vi "HEWH Get FHD.vi"(7 "Water Heater Type":T1, 8 "error in (no error)":errorcluster, 10 "FHD During 1 Hour Input":T2 {"Data Indexes"."15 sec after Draw Index" format="%#.2f"; "Data Indexes"."15 sec after Draw Timestamp" format="%#.2f"; "Data Indexes"."Test Start Timestamp" format="%.2f"; "Data Indexes"."Test End Timestamp" format="%.2f"; "Data Indexes"."T0 Timestamp" format="%.2f"; "Data Indexes"."Tsf Timestamp" format="%.2f"; "Data Indexes"."Tsu0 Timestamp" format="%.2f"; "Data Indexes"."Tmax1 Timestamp" format="%.2f"; "Data Indexes"."Draw Index Timestamp" format="%#.2f"; "Data Indexes"."Non-Draw Timestamp" format="%#.2f"; "Data Indexes"."Heating Timestamp" format="%#.2f"; "Data Indexes"."Start Energy (BTU-Gas)" format="%.6f"; "Data Indexes"."Start Watt Hours" format="%.6f"; "Static Data"."V - Volume of Wh (True)" format="%.5f"; "Static Data"."T-Ambinet Nominal (°F)" format="%.5f"; "Static Data"."T-Inlet Setpoint (°F)" format="%.5f"; "Static Data"."T-Wh Setpoint (°F)" format="%.5f"; "Sampled Data"."Qe (Wh)" format="%.5f"; "Sampled Data"."Tau stby2 (hr)" format="%.5f"; "Sampled Data"."Tastby2 (°F)" format="%.5f"; "Sampled Data"."Qf (BTU)" format="%.5f"; "Sampled Data"."Qe (BTU)" format="%.5f"; "Sampled Data"."Tmax1 (°F)" format="%.5f"; "Sampled Data"."T0 (°F)" format="%.5f"; "Sampled Data"."Qr (BTU)" format="%.5f"; "Sampled Data"."T 24(°F)" format="%.5f"; "Sampled Data"."T astby(°F)" format="%.5f"; "Sampled Data"."T tstby(°F)" format="%.5f"; "Sampled Data"."T su0(°F)" format="%.5f"; "Sampled Data"."T suf(°F)" format="%.5f"; "Sampled Data"."Tau stby_1 (hr)" format="%.5f"; "Sampled Data"."Qsuf (BTU)" format="%.5f"; "Sampled Data"."Qsu0 (BTU)" format="%.5f"; "Calculated Values"."Draw Bonus Volume (gal)" format="%.6f"; "Calculated Values"."Adjustment Factor" format="%.6f"; "Calculated Values"."T*avg_del(n-1)" format="%.6f"; "Calculated Values"."T*min(n-1)" format="%.6f"; "Calculated Values"."T*avg_del(n)" format="%.6f"; "Calculated Values"."Vn" format="%.6f"; "Calculated Values"."Qdm (BTU)" format="%.6f"; "Calculated Values"."QHWD (BTU)" format="%.6f"; "Calculated Values"."QHW (BTU)" format="%.6f"; "Calculated Values"."UEF" format="%.6f"; "Calculated Values"."QHW67 (BTU)" format="%.6f"; "Calculated Values"."Qda (BTU)" format="%.6f"; "Calculated Values"."Qd (BTU)" format="%.6f"; "Calculated Values"."Q (BTU)" format="%.6f"; "Calculated Values"."UA (BTU/(hr*F))" format="%.6f"; "Calculated Values"."Qhr (BTU/hr)" format="%.6f"; "Calculated Values"."Qstby (BTU)" format="%.6f"; "Calculated Values"."nu_r" format="%.6f"; "Calculated Values"."CpUEF (BTU/(lb*F))" format="%.6f"; "Calculated Values"."rho_nu (lb/gal)" format="%.6f"; "Calculated Values"."V1- Vol (Gal)" format="%.6f"; "Calculated Values"."M cluster mass removed (lb)" format="%.6f"; "Calculated Values"."Cp theoretical (BTU/(lbm °F))" format="%.6f"; "Calculated Values"."Tin1 - Mean Inlet 1st Cluster (°F)" format="%.6f"; "Calculated Values"."Tdel1-Mean Outlet 1st Cluster(°F)" format="%.6f"; "Calculated Values"."Cp 24 (BTU/(lb*F))" format="%.6f"; "Calculated Values"."Cp standby (BTU/(lb*F))" format="%.6f"; "Calculated Values"."Cp2 (BTU/(lb*F))" format="%.6f"; "Calculated Values"."Cp1 (BTU/(lb*F))" format="%.6f"; "Calculated Values"."rho 24 (lb/gal)" format="%.6f"; "Calculated Values"."rho standby (lb/gal)" format="%.6f"; "Calculated Values"."rho 2 (lb/gal)" format="%.6f"; "Calculated Values"."Density of cold water All (lbm/gal)" format="%#.3g"; "Calculated Values"."CpHW (BTU/(lbm °F))" format="%#.3g"; "Calculated Values"."Density of hot water All (lbm/gal)" format="%#.3g"; "Calculated Values"."Mass of water All (lbm)" format="%#.3f"}, 11 "1st Hour Location":path) -> (0 "error out":errorcluster, 1 "First Hour Rating (Gallons)":dbl, 2 "FHD During 1 Hour Output":T2={"Calculated Values"={"Draw Cluster - Actual (Gal)"=[], "Mass of water All (lbm)"=[], "Density of hot water All (lbm/gal)"=[], "CpHW (BTU/(lbm °F))"=[], "rho 2 (lb/gal)"=0.0, "rho standby (lb/gal)"=0.0, "rho 24 (lb/gal)"=0.0, "Cp1 (BTU/(lb*F))"=0.0, "Cp2 (BTU/(lb*F))"=0.0, "Cp standby (BTU/(lb*F))"=0.0, "Cp 24 (BTU/(lb*F))"=0.0, "nu_r"=0.0, "Qstby (BTU)"=0.0, "Qhr (BTU/hr)"=0.0, "UA (BTU/(hr*F))"=0.0, "Q (BTU)"=0.0, "Qd (BTU)"=0.0, "Qda (BTU)"=0.0, "QHW67 (BTU)"=0.0, "UEF"=0.0, "Tdel1-Mean Outlet 1st Cluster(°F)"=0.0, "Tin1 - Mean Inlet 1st Cluster (°F)"=0.0, "Cp theoretical (BTU/(lbm °F))"=0.0, "M cluster mass removed (lb)"=0.0, "V1- Vol (Gal)"=0.0, "Test Data -Start to End (Full Index)"=[], "rho_nu (lb/gal)"=0.0, "Density of cold water All (lbm/gal)"=[], "CpUEF (BTU/(lb*F))"=0.0, "QHW (BTU)"=0.0, "QHWD (BTU)"=0.0, "Qdm (BTU)"=0.0, "FHD-After 1 Hour (String)"=[], "Vn"=0.0, "T*avg_del(n)"=0.0, "Max Location"=0, "T*min(n-1)"=0.0, "T*avg_del(n-1)"=0.0, "Temp Greater than T*min(n-1)"=FALSE, "Adjustment Factor"=0.0, "Draw Bonus Volume (gal)"=0.0, "Flow Type - End Condition"=enum."ForcedDrawAfterHour"}, "Sampled Data"={"Cold Water Draw Amounts-(Gal)"=[14.98, 1.97, 9.0, 8.97, 4.98, 0.98, 0.96, 0.96, 0.96, 1.96, 1.99, 6.98], "T del_all - Outlet Temps (°F)"=[121.5, 121.3, 124.5, 120.0, 121.2, 120.1, 119.0, 120.3, 116.6, 118.8, 118.3, 118.3], "T in_all - Inlet Temps (°F)"=[58.5, 58.2, 58.4, 58.6, 58.6, 58.1, 58.1, 58.3, 56.3, 58.5, 58.5, 58.5], "Qsu0 (BTU)"=9772.3, "Qsuf (BTU)"=9773.0, "Tau stby_1 (hr)"=6.7, "T suf(°F)"=107.7, "T su0(°F)"=109.3, "T tstby(°F)"=108.5, "T astby(°F)"=68.2, "T 24(°F)"=117.9, "Qr (BTU)"=7628.5, "T0 (°F)"=121.1, "Tmax1 (°F)"=122.4, "Qe (BTU)"=29606.3, "Qf (BTU)"=0.0, "Tastby2 (°F)"=68.3, "RTD Out Full Data\nSet (Each Draw)"=[], "RTD IN Full Data\nSet (Each Draw)"=[], "Tau stby2 (hr)"=23.406, "Hot Water Draw Amounts-(Gal)"=[], "Cold Flow Rate (GPM)"=[], "Hot Flow Rate (GPM)"=[], "Softw Elapsed Time\n Full Data Set (Each Draw)"=[], "Cold Gal Total Full\nData Set (Each Draw)"=[], "Total Hot Draw Amount (Gal) "=0.0, "Total Cold Draw Amount (Gal)"=0.0, "Qe (Wh)"=0.0, "Hot Gal Total Full\nData Set (Each Draw)"=[]}, "Static Data"={"T-Wh Setpoint (°F)"=125.0, "T-Inlet Setpoint (°F)"=58.0, "T-Ambinet Nominal (°F)"=67.5, "V - Volume of Wh (True)"=46.0}, "Data Indexes"={"Test Start-Full Index (Found)"=0, "Header Length"=0, "Draw Index (Found)"=[], "Nr"=0, "Start Watt Hours"=0.0, "Tsu0 Index (Found)"=0, "Tsf Index (Found)"=0, "Start Energy (BTU-Gas)"=0.0, "Draws in Cluster"=0, "T0 Index-Full Index (Found)"=0, "Non-Draw Index (Found)"=[], "Tmax1 Index (Found)"=0, "Test End-Full Index (Found)"=0, "Heating Index (Found)"=[], "Heating Timestamp"=[], "Non-Draw Timestamp"=[], "Draw Index Timestamp"=[], "Tmax1 Timestamp"=0.0, "Tsu0 Timestamp"=0.0, "Tsf Timestamp"=0.0, "T0 Timestamp"=0.0, "Test End Timestamp"=0.0, "Test Start Timestamp"=0.0, "15 sec after Draw Timestamp"=[], "15 sec after Draw Index"=[], "Tmax1 Occurred During a Draw"=FALSE, "FHD Total Time (Sec)"=0.0, "Draw Pattern"=enum."Very Small Usage", "Standby Valid"=FALSE}, "Raw Data"={"Elapsed Time Index (DBL)"=0, "Software Elapsed Time Index (DBL)"=0, "TC Tree Avg Index (DBL)"=0, "Watt Hours -Wh Index (DBL)"=0, "Energy BTU Index (DBL)"=0, "Totalized Flow Index (DBL)"=0, "Flow Rate Index (DBL)"=0, "Program Status Index (Str)"=0, "RTDin Index (DBL)"=0, "RTDout Index (DBL)"=0, "RTDamb Index (DBL)"=0, "Test Data-Start to End DBL"=[], "Data Type"=enum."GEA Inlet Side Meter", "Heat Source Index (DBL)"=0, "Hot Water Rate GPM (DBL)"=0, "Hot Water Total - GAL (DBL)"=0, "FHD-After 1 hour"=[], "Humidity -% RH (DBL)"=0, "Voltage - V (DBL)"=0, "Draw Count (DBL)"=0, "Elapsed Time Index (Str)"=0, "Software Elapsed Time Index (Str)"=0, "Frequency-Hz (Str)"=0, "RTDin Index (Str)"=0, "RTDout Index (Str)"=0, "RTDamb Index (Str)"=0, "UE (Str)"=0, "LE (Str)"=0, "Compressor (Str)"=0, "Flow Rate Index (Str)"=0, "Hot Water Total - GAL (Str)"=0}, "Tolerance Check (T)=Pass"={"Flow Rate"=FALSE, "Totalized Flow"=FALSE, "Ambient Temp (Full Range)"=FALSE, "Ambient Humidity (Full Range)"=FALSE, "Inlet Temp"=FALSE, "Outlet Temp"=FALSE, "Valid Test"=FALSE, "Individual Totalized Flow"=FALSE, "Data Sheet Check"="", "Inlet Temperature"=[], "Tinlet Max"=[], "Tinlet Min"=[], "Flow Rate Max (Tol)"=[], "Flow Rate Min (Tol)"=[], "Amb Temp Max"=0.0, "Amb Temp Min"=0.0, "Toutlet Max - Draw 1"=0.0, "Humidity Upper Tolerance (%)"=0.0, "Total Volume Tolerance (Gal)"=0.0, "Humidity Lower Tolerance (%)"=0.0, "Flow Rate Max\nPer Draw"=[], "Flow Rate Min\nPer Draw"=[], "Ambient Humidity (Runtime)"=FALSE, "Humidity Avg (Runtime)"=0.0, "Ambient Temp (On-Time AVG)"=FALSE, "Ambient Temp (Off-Time AVG)"=FALSE, "Amb Temp OFF Avg"=0.0, "Amb Temp ON Avg"=0.0, "Voltage (Heating)"=FALSE, "Voltage (Min)"=0.0, "Voltage (Max)"=0.0, "Toutlet Max"=[], "Toutlet Min"=[], "Test_Avg_Outlet_Temp"=0.0}, "Test Information"={"TR Number"="", "Lab ID"="", "Notes/Config"="", "Model Number"="", "Serial Number"="", "Lab Technician"="", "Engineer"="", "Type of Fuel"="", "Samp Received Date"="", "Samp Test Date"="", "Report Date"="", "Rate Input (kW or BTU/hr)"="", "Measured Input (kW or BTU/hr)"="", "Filename"="", "Calibration Information"=[], "Calculator Version"="", "Minimum UEF Per CFR"=0.0, "UEF Report Information"=[], "FHR Report Information"=[], "FHR Front Panel Display"=[], "UEF Front Panel Display"=[], "Draw Outlet Temp Viewer"=[]}} {"Data Indexes"."15 sec after Draw Index" format="%#.2f"; "Data Indexes"."15 sec after Draw Timestamp" format="%#.2f"; "Data Indexes"."Test Start Timestamp" format="%.2f"; "Data Indexes"."Test End Timestamp" format="%.2f"; "Data Indexes"."T0 Timestamp" format="%.2f"; "Data Indexes"."Tsf Timestamp" format="%.2f"; "Data Indexes"."Tsu0 Timestamp" format="%.2f"; "Data Indexes"."Tmax1 Timestamp" format="%.2f"; "Data Indexes"."Draw Index Timestamp" format="%#.2f"; "Data Indexes"."Non-Draw Timestamp" format="%#.2f"; "Data Indexes"."Heating Timestamp" format="%#.2f"; "Data Indexes"."Start Energy (BTU-Gas)" format="%.6f"; "Data Indexes"."Start Watt Hours" format="%.6f"; "Static Data"."V - Volume of Wh (True)" format="%.5f"; "Static Data"."T-Ambinet Nominal (°F)" format="%.5f"; "Static Data"."T-Inlet Setpoint (°F)" format="%.5f"; "Static Data"."T-Wh Setpoint (°F)" format="%.5f"; "Sampled Data"."Qe (Wh)" format="%.5f"; "Sampled Data"."Tau stby2 (hr)" format="%.5f"; "Sampled Data"."Tastby2 (°F)" format="%.5f"; "Sampled Data"."Qf (BTU)" format="%.5f"; "Sampled Data"."Qe (BTU)" format="%.5f"; "Sampled Data"."Tmax1 (°F)" format="%.5f"; "Sampled Data"."T0 (°F)" format="%.5f"; "Sampled Data"."Qr (BTU)" format="%.5f"; "Sampled Data"."T 24(°F)" format="%.5f"; "Sampled Data"."T astby(°F)" format="%.5f"; "Sampled Data"."T tstby(°F)" format="%.5f"; "Sampled Data"."T su0(°F)" format="%.5f"; "Sampled Data"."T suf(°F)" format="%.5f"; "Sampled Data"."Tau stby_1 (hr)" format="%.5f"; "Sampled Data"."Qsuf (BTU)" format="%.5f"; "Sampled Data"."Qsu0 (BTU)" format="%.5f"; "Calculated Values"."Draw Bonus Volume (gal)" format="%.6f"; "Calculated Values"."Adjustment Factor" format="%.6f"; "Calculated Values"."T*avg_del(n-1)" format="%.6f"; "Calculated Values"."T*min(n-1)" format="%.6f"; "Calculated Values"."T*avg_del(n)" format="%.6f"; "Calculated Values"."Vn" format="%.6f"; "Calculated Values"."Qdm (BTU)" format="%.6f"; "Calculated Values"."QHWD (BTU)" format="%.6f"; "Calculated Values"."QHW (BTU)" format="%.6f"; "Calculated Values"."UEF" format="%.6f"; "Calculated Values"."QHW67 (BTU)" format="%.6f"; "Calculated Values"."Qda (BTU)" format="%.6f"; "Calculated Values"."Qd (BTU)" format="%.6f"; "Calculated Values"."Q (BTU)" format="%.6f"; "Calculated Values"."UA (BTU/(hr*F))" format="%.6f"; "Calculated Values"."Qhr (BTU/hr)" format="%.6f"; "Calculated Values"."Qstby (BTU)" format="%.6f"; "Calculated Values"."nu_r" format="%.6f"; "Calculated Values"."CpUEF (BTU/(lb*F))" format="%.6f"; "Calculated Values"."rho_nu (lb/gal)" format="%.6f"; "Calculated Values"."V1- Vol (Gal)" format="%.6f"; "Calculated Values"."M cluster mass removed (lb)" format="%.6f"; "Calculated Values"."Cp theoretical (BTU/(lbm °F))" format="%.6f"; "Calculated Values"."Tin1 - Mean Inlet 1st Cluster (°F)" format="%.6f"; "Calculated Values"."Tdel1-Mean Outlet 1st Cluster(°F)" format="%.6f"; "Calculated Values"."Cp 24 (BTU/(lb*F))" format="%.6f"; "Calculated Values"."Cp standby (BTU/(lb*F))" format="%.6f"; "Calculated Values"."Cp2 (BTU/(lb*F))" format="%.6f"; "Calculated Values"."Cp1 (BTU/(lb*F))" format="%.6f"; "Calculated Values"."rho 24 (lb/gal)" format="%.6f"; "Calculated Values"."rho standby (lb/gal)" format="%.6f"; "Calculated Values"."rho 2 (lb/gal)" format="%.6f"; "Calculated Values"."Density of cold water All (lbm/gal)" format="%#.3g"; "Calculated Values"."CpHW (BTU/(lbm °F))" format="%#.3g"; "Calculated Values"."Density of hot water All (lbm/gal)" format="%#.3g"; "Calculated Values"."Mass of water All (lbm)" format="%#.3f"}, 4 "FHD Full Data":string[][](array[string]), 6 "PercentInRange":dbl)   [LabVIEW 2023]
uses:
  Type Definitions/UEF Constants.ctl
  Type Definitions/HEWH Draw Stats.ctl
  Type Definitions/HEWH FHR Draw Type.ctl
  Type Definitions/FHR Bins.ctl
  Type Definitions/HEWH Meter Type.ctl
  Type Definitions/HEWH Water Heater Type.ctl
  Type Definitions/HEWH Test Type.ctl
  Type Definitions/HEWH Index Type.ctl
  <vilib>/Utility/file.llb/Read Delimited Spreadsheet (string).vi
  <vilib>/Utility/file.llb/Read Delimited Spreadsheet (DBL).vi
panel:
  # "FHR"
  # "FHR"
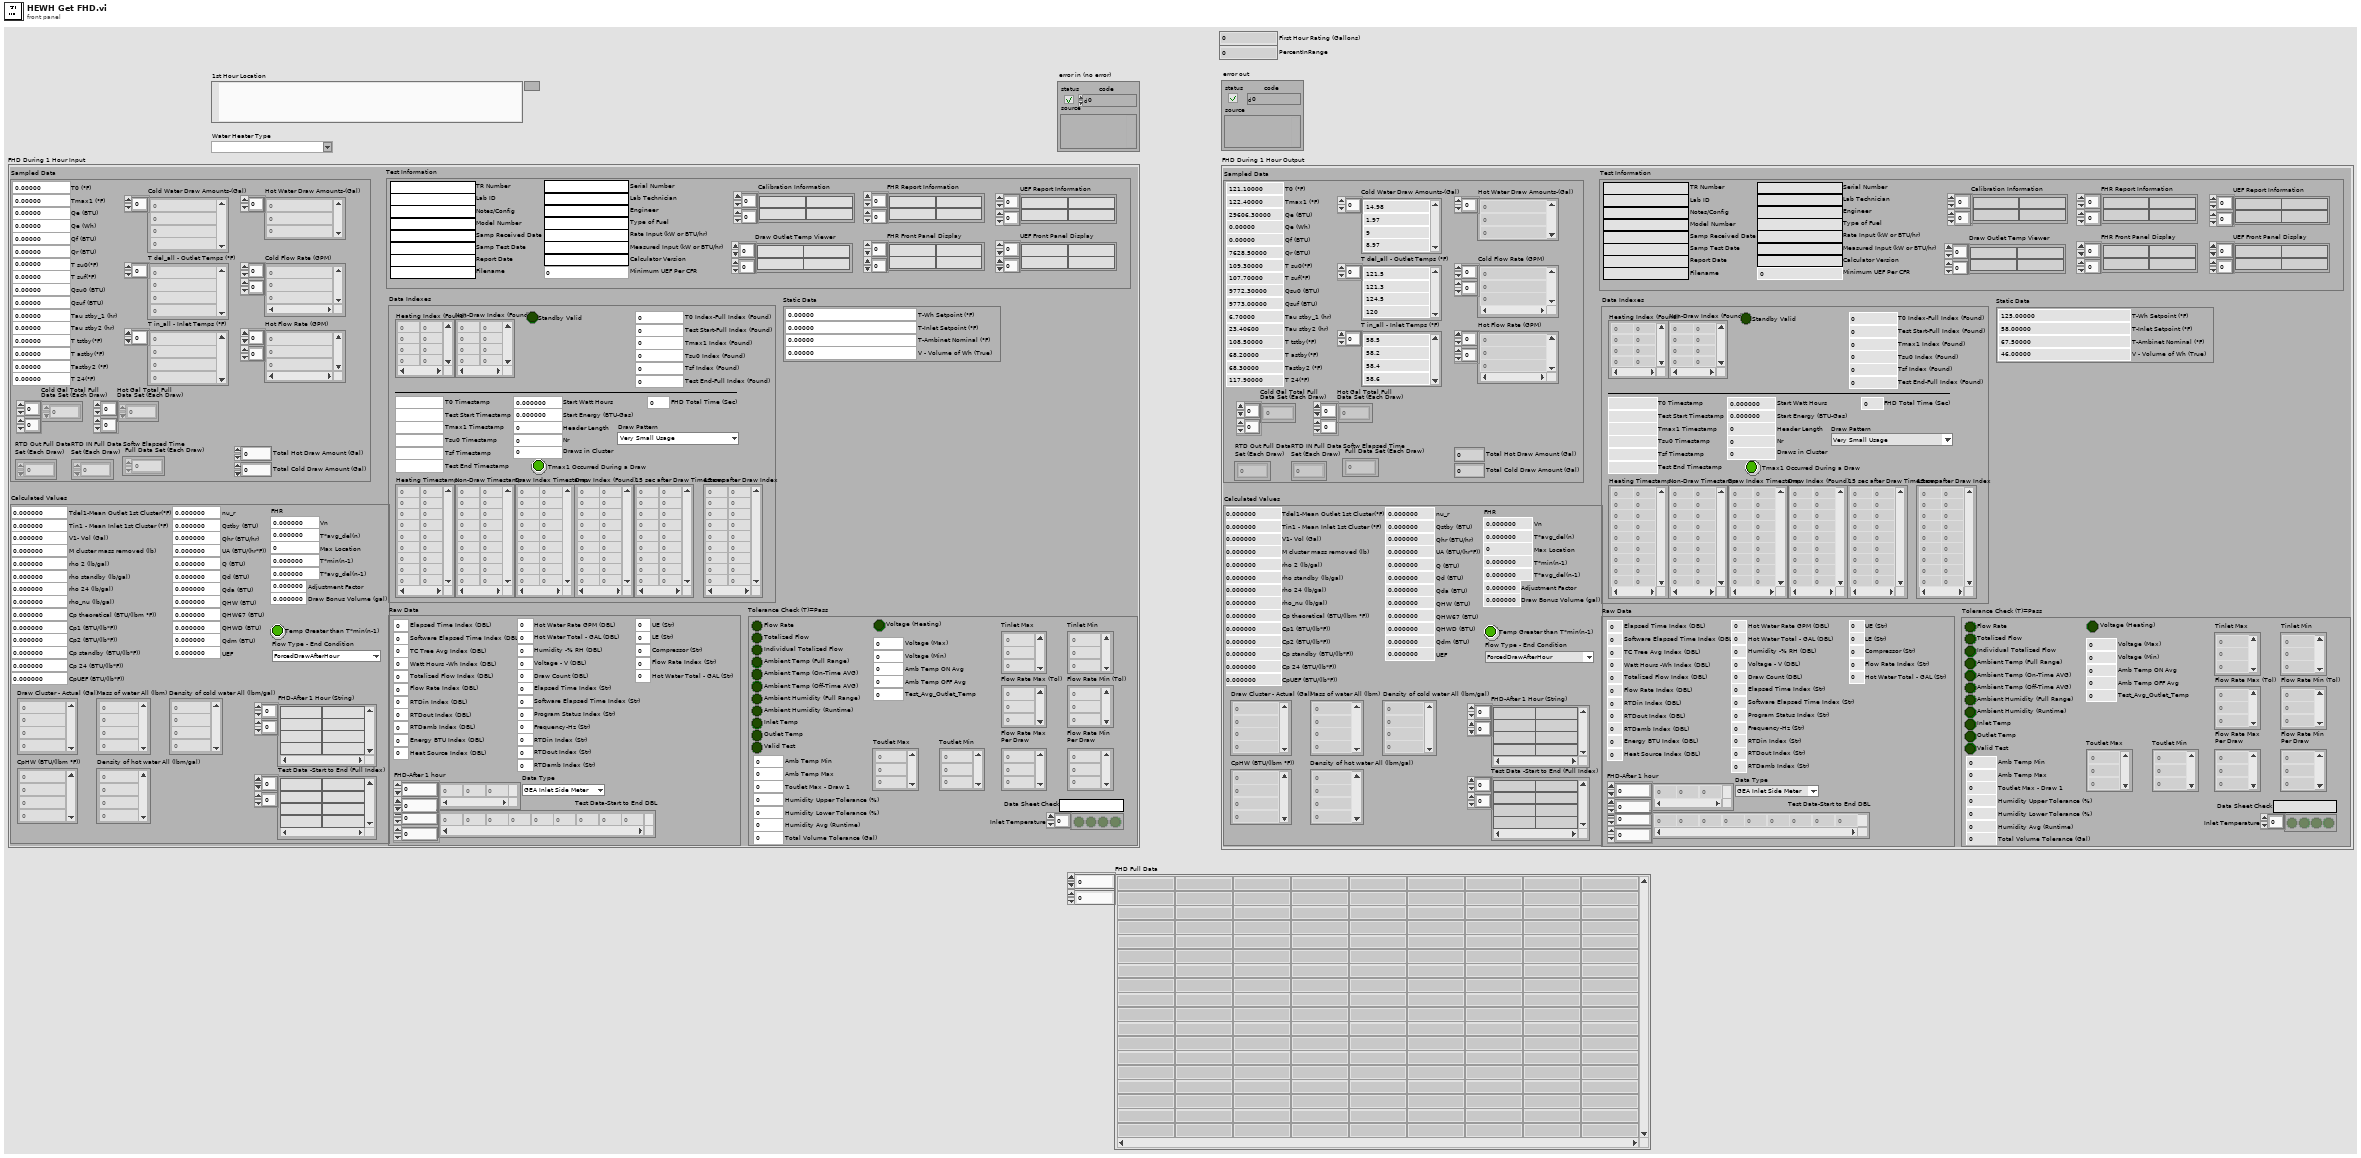
[diagram p1: front panel]
types:
  T1 = typedef "HEWH Water Heater Type.ctl" = string
  T2 = typedef "UEF Constants.ctl" = cluster{"Calculated Values":T3, "Sampled Data":cluster{"Cold Water Draw Amounts-(Gal)":dbl[], "T del_all - Outlet Temps (°F)":dbl[], "T in_all - Inlet Temps (°F)":dbl[], "Qsu0 (BTU)":dbl, "Qsuf (BTU)":dbl, "Tau stby_1 (hr)":dbl, "T suf(°F)":dbl, "T su0(°F)":dbl, "T tstby(°F)":dbl, "T astby(°F)":dbl, "T 24(°F)":dbl, "Qr (BTU)":dbl, "T0 (°F)":dbl, "Tmax1 (°F)":dbl, "Qe (BTU)":dbl, "Qf (BTU)":dbl, "Tastby2 (°F)":dbl, "RTD Out Full Data\nSet (Each Draw)":dbl[][], "RTD IN Full Data\nSet (Each Draw)":dbl[][], "Tau stby2 (hr)":dbl, "Hot Water Draw Amounts-(Gal)":dbl[], "Cold Flow Rate (GPM)":dbl[][], "Hot Flow Rate (GPM)":dbl[][], "Softw Elapsed Time\n Full Data Set (Each Draw)":dbl[][], "Cold Gal Total Full\nData Set (Each Draw)":dbl[][], "Total Hot Draw Amount (Gal) ":dbl, "Total Cold Draw Amount (Gal)":dbl, "Qe (Wh)":dbl, "Hot Gal Total Full\nData Set (Each Draw)":dbl[][]}, "Static Data":cluster{"T-Wh Setpoint (°F)":dbl, "T-Inlet Setpoint (°F)":dbl, "T-Ambinet Nominal (°F)":dbl, "V - Volume of Wh (True)":dbl}, "Data Indexes":cluster{"Test Start-Full Index (Found)":i32, "Header Length":i32, "Draw Index (Found)":i32[][], "Nr":i32, "Start Watt Hours":dbl, "Tsu0 Index (Found)":i32, "Tsf Index (Found)":i32, "Start Energy (BTU-Gas)":dbl, "Draws in Cluster":i32, "T0 Index-Full Index (Found)":i32, "Non-Draw Index (Found)":i32[][], "Tmax1 Index (Found)":i32, "Test End-Full Index (Found)":i32, "Heating Index (Found)":i32[][], "Heating Timestamp":dbl[][], "Non-Draw Timestamp":dbl[][], "Draw Index Timestamp":dbl[][], "Tmax1 Timestamp":dbl, "Tsu0 Timestamp":dbl, "Tsf Timestamp":dbl, "T0 Timestamp":dbl, "Test End Timestamp":dbl, "Test Start Timestamp":dbl, "15 sec after Draw Timestamp":dbl[][], "15 sec after Draw Index":dbl[][], "Tmax1 Occurred During a Draw":bool, "FHD Total Time (Sec)":dbl, "Draw Pattern":T5, "Standby Valid":bool}, "Raw Data":cluster{"Elapsed Time Index (DBL)":i32, "Software Elapsed Time Index (DBL)":i32, "TC Tree Avg Index (DBL)":i32, "Watt Hours -Wh Index (DBL)":i32, "Energy BTU Index (DBL)":i32, "Totalized Flow Index (DBL)":i32, "Flow Rate Index (DBL)":i32, "Program Status Index (Str)":i32, "RTDin Index (DBL)":i32, "RTDout Index (DBL)":i32, "RTDamb Index (DBL)":i32, "Test Data-Start to End DBL":dbl[][], "Data Type":T6, "Heat Source Index (DBL)":i32, "Hot Water Rate GPM (DBL)":i32, "Hot Water Total - GAL (DBL)":i32, "FHD-After 1 hour":dbl[][], "Humidity -% RH (DBL)":i32, "Voltage - V (DBL)":i32, "Draw Count (DBL)":i32, "Elapsed Time Index (Str)":i32, "Software Elapsed Time Index (Str)":i32, "Frequency-Hz (Str)":i32, "RTDin Index (Str)":i32, "RTDout Index (Str)":i32, "RTDamb Index (Str)":i32, "UE (Str)":i32, "LE (Str)":i32, "Compressor (Str)":i32, "Flow Rate Index (Str)":i32, "Hot Water Total - GAL (Str)":i32}, "Tolerance Check (T)=Pass":cluster{"Flow Rate":bool, "Totalized Flow":bool, "Ambient Temp (Full Range)":bool, "Ambient Humidity (Full Range)":bool, "Inlet Temp":bool, "Outlet Temp":bool, "Valid Test":bool, "Individual Totalized Flow":bool, "Data Sheet Check":string, "Inlet Temperature":bool[], "Tinlet Max":dbl[], "Tinlet Min":dbl[], "Flow Rate Max (Tol)":dbl[], "Flow Rate Min (Tol)":dbl[], "Amb Temp Max":dbl, "Amb Temp Min":dbl, "Toutlet Max - Draw 1":dbl, "Humidity Upper Tolerance (%)":dbl, "Total Volume Tolerance (Gal)":dbl, "Humidity Lower Tolerance (%)":dbl, "Flow Rate Max\nPer Draw":dbl[], "Flow Rate Min\nPer Draw":dbl[], "Ambient Humidity (Runtime)":bool, "Humidity Avg (Runtime)":dbl, "Ambient Temp (On-Time AVG)":bool, "Ambient Temp (Off-Time AVG)":bool, "Amb Temp OFF Avg":dbl, "Amb Temp ON Avg":dbl, "Voltage (Heating)":bool, "Voltage (Min)":dbl, "Voltage (Max)":dbl, "Toutlet Max":dbl[], "Toutlet Min":dbl[], "Test_Avg_Outlet_Temp":dbl}, "Test Information":cluster{"TR Number":string, "Lab ID":string, "Notes/Config":string, "Model Number":string, "Serial Number":string, "Lab Technician":string, "Engineer":string, "Type of Fuel":string, "Samp Received Date":string, "Samp Test Date":string, "Report Date":string, "Rate Input (kW or BTU/hr)":string, "Measured Input (kW or BTU/hr)":string, "Filename":string, "Calibration Information":string[][], "Calculator Version":string, "Minimum UEF Per CFR":dbl, "UEF Report Information":string[][], "FHR Report Information":string[][], "FHR Front Panel Display":string[][], "UEF Front Panel Display":string[][], "Draw Outlet Temp Viewer":string[][]}}
  T3 = typedef "HEWH Draw Stats.ctl" = cluster{"Draw Cluster - Actual (Gal)":dbl[], "Mass of water All (lbm)":dbl[], "Density of hot water All (lbm/gal)":dbl[], "CpHW (BTU/(lbm °F))":dbl[], "rho 2 (lb/gal)":dbl, "rho standby (lb/gal)":dbl, "rho 24 (lb/gal)":dbl, "Cp1 (BTU/(lb*F))":dbl, "Cp2 (BTU/(lb*F))":dbl, "Cp standby (BTU/(lb*F))":dbl, "Cp 24 (BTU/(lb*F))":dbl, "nu_r":dbl, "Qstby (BTU)":dbl, "Qhr (BTU/hr)":dbl, "UA (BTU/(hr*F))":dbl, "Q (BTU)":dbl, "Qd (BTU)":dbl, "Qda (BTU)":dbl, "QHW67 (BTU)":dbl, "UEF":dbl, "Tdel1-Mean Outlet 1st Cluster(°F)":dbl, "Tin1 - Mean Inlet 1st Cluster (°F)":dbl, "Cp theoretical (BTU/(lbm °F))":dbl, "M cluster mass removed (lb)":dbl, "V1- Vol (Gal)":dbl, "Test Data -Start to End (Full Index)":string[][], "rho_nu (lb/gal)":dbl, "Density of cold water All (lbm/gal)":dbl[], "CpUEF (BTU/(lb*F))":dbl, "QHW (BTU)":dbl, "QHWD (BTU)":dbl, "Qdm (BTU)":dbl, "FHD-After 1 Hour (String)":string[][], "Vn":dbl, "T*avg_del(n)":dbl, "Max Location":i32, "T*min(n-1)":dbl, "T*avg_del(n-1)":dbl, "Temp Greater than T*min(n-1)":bool, "Adjustment Factor":dbl, "Draw Bonus Volume (gal)":dbl, "Flow Type - End Condition":T4}
  T4 = typedef "HEWH FHR Draw Type.ctl" = enum16{"ForcedDrawAfterHour", "HeatingCutoffBeforeHour"}
  T5 = typedef "FHR Bins.ctl" = enum16{"Very Small Usage", "Low Usage", "Medium Usage", "High Usage", "Undefined"}
  T6 = typedef "HEWH Meter Type.ctl" = enum16{"GEA Inlet Side Meter", "GEA Outlet Side Meter", "CSA Inlet Side Meter"}
  T7 = typedef "HEWH Index Type.ctl" = enum16{"Draw Index", "Heating Index", "Temp Based (FHD)"}
  T8 = typedef "HEWH Test Type.ctl" = enum16{"UEF", "FHD"}
  T9 = typedef "Upper Most Element.ctl" = enum16{"Compressor", "Lower Element", "Upper Element"}
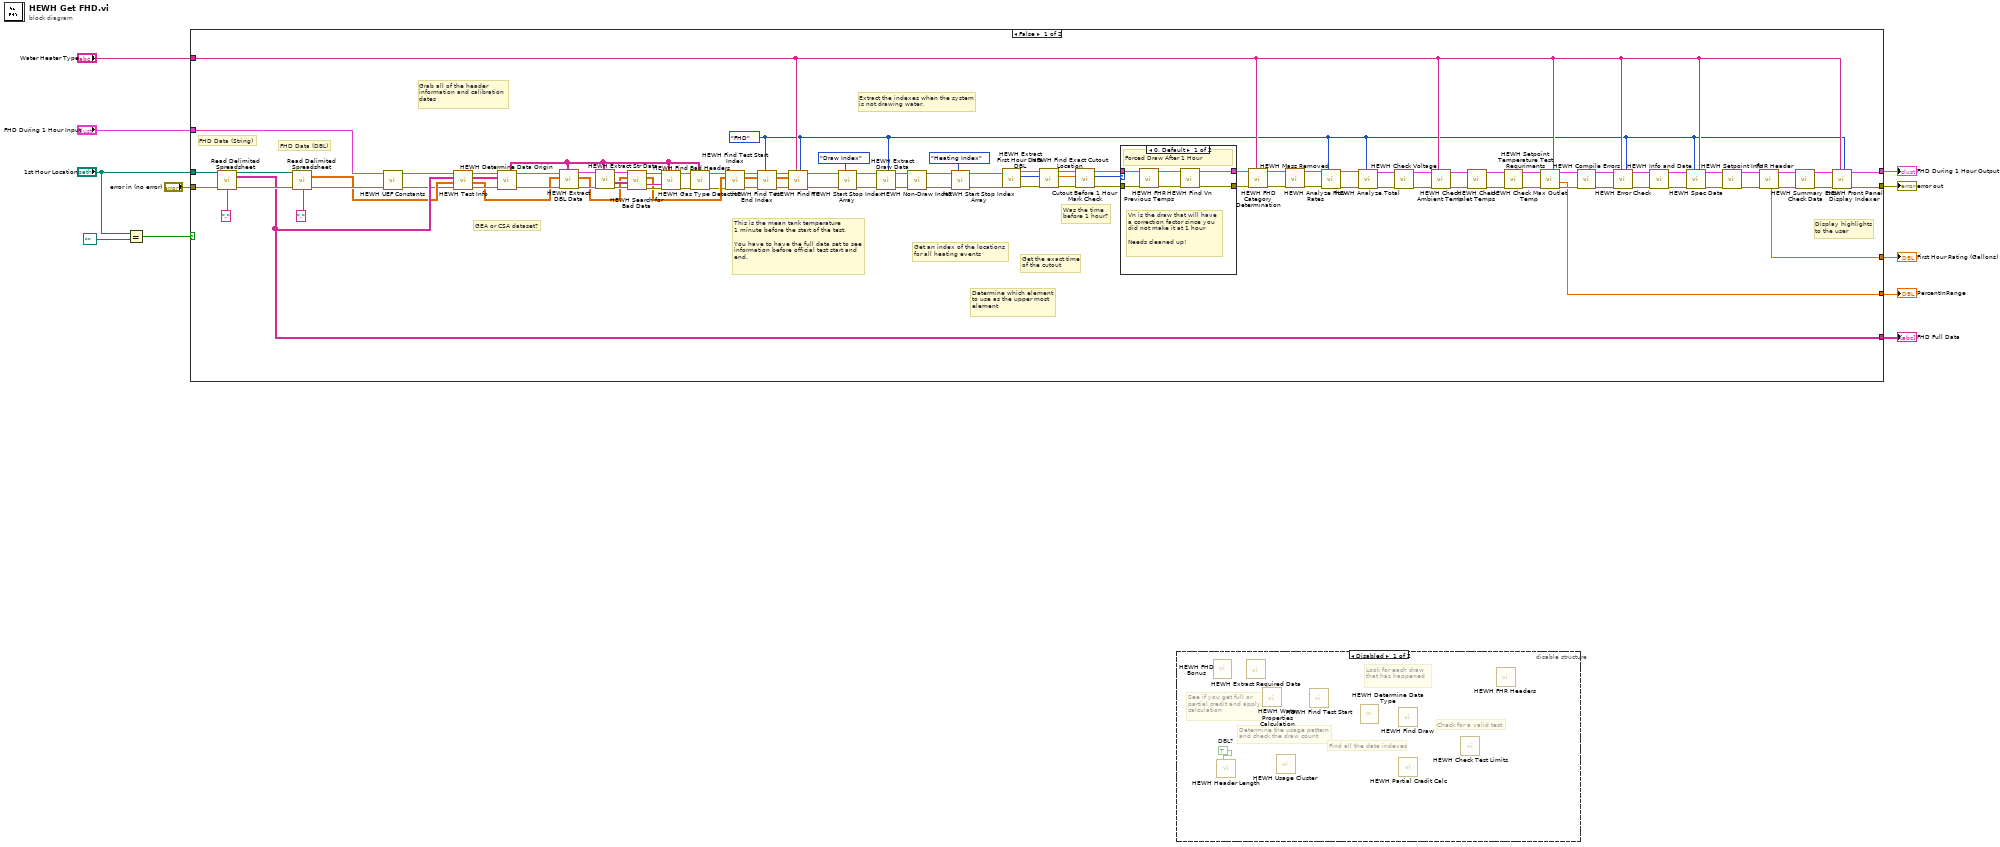
[diagram p0: block diagram]
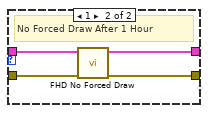
[diagram p3: hidden frame]
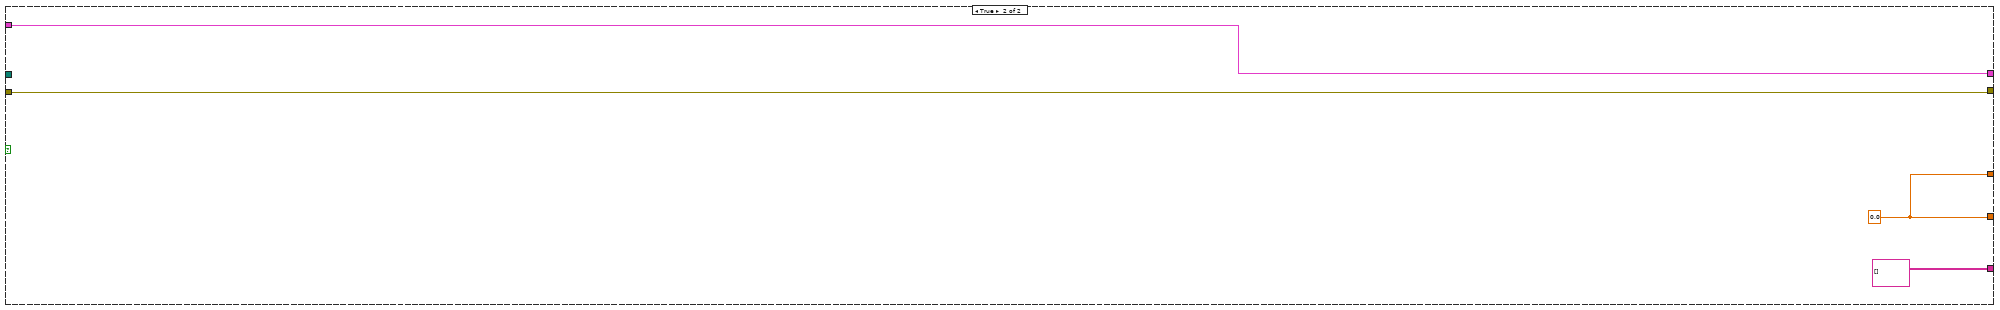
[diagram p4: hidden frame]
diagram:
  n1 = Equal?(x="1st Hour Location", y=path "") -> (x = y?=w4:bool)
  n2 = case shown="False" w4 {
    tunnel: "FHD During 1 Hour Input" -> [w85 w125]
    tunnel: [w56 string[][] [] ("all rows")] -> w10
    tunnel: "Water Heater Type" -> [w19 _]
    tunnel: "1st Hour Location" -> [w108 _]
    tunnel: "error in (no error)" -> [w106 w124]
    tunnel: [w14 w125] -> w2
    tunnel: [w105 w124] -> w7
    tunnel: [w18 w122] -> w3
    tunnel: [w13 w122] -> w1
    frame False {
      w12 = HEWH_Test_Type."FHD" ("Test Type")
      # "Get an index of the locations \nfor all heating events"
      # "Extract the indexes when the system\nis not drawing water."
      # "GEA or CSA dataset?"
      # "Grab all of the header\ninformation and calibration\ndates"
      # "This is the mean tank temperature\n1 minute before the start of the test.\n\nYou have to have the full data set to see\ninformation before official test start and \nend."
      # "Was the time\nbefore 1 hour?"
      # "Get the exact time\nof the cutout"
      # "Determine which element\nto use as the upper most\nelement"
      # "Display highlights\nto the user"
      # "FHD Data (String)"
      # "FHD Data (DBL)"
      n3 = call-poly <vilib>:"Read Delimited Spreadsheet.vi"("file path (dialog if empty)"=w108, "error in (no error)"=w106, "delimiter (\\t)"="," ("delimiter (\\t)")) -> ("new file path (Not A Path if cancelled)"=w109:path, "all rows"=w56:string[][], "error out"=w107:errorcluster)  [unwired: 7 in, 3 out]
      n4 = call-poly <vilib>:"Read Delimited Spreadsheet.vi"("file path (dialog if empty)"=w109, "error in (no error)"=w107, "delimiter (\\t)"="," ("delimiter (\\t)")) -> ("all rows"=w52:dbl[][], "error out"=w84:errorcluster)  [unwired: 7 in, 4 out]
      n5 = call "HEWH UEF Constants.vi"("error in (no error)"=w84, "UEF Calculated Values Input"=w85) -> ("error out"=w50:errorcluster, "UEF Calculated Values Output"=w57:T2)  [unwired: 8 in]
      n6 = call "HEWH Test Info.vi"("error in (no error)"=w50, "Full Data DBL"=w52, "Full Data (String)"=w56, "UEF Calculated Values Input"=w57) -> ("error out"=w53:errorcluster, "Full Data DBL Out"=w51:dbl[][], "Full Data (String)"=w54:string[][], "UEF Calculated Values Output"=w55:T2)  [unwired: 4 in]
      n7 = call "HEWH Determine Data Origin.vi"("error in (no error)"=w53, "Full Data (String)"=w54, "UEF Calculated Values Output in"=w55) -> ("error out"=w58:errorcluster, "UEF Calculated Values Output out"=w59:T2, "Full Data (String) Out"=w60:string[][])  [unwired: 6 in]
      n8 = call "HEWH Extract DBL Data.vi"("Full Data (String)"=w60, "error in (no error)"=w58, "Full Data DBL In"=w51, "UEF Calculated Values Input in"=w59) -> ("error out"=w68:errorcluster, "Full Data DBL Out"=w65:dbl[][], "UEF Calculated Values Input out"=w71:T2)  [unwired: 5 in]
      n9 = call "HEWH Extract Str Data.vi"("Full Data (String)"=w60, "error in (no error)"=w68, "UEF Calculated Values Input in"=w71) -> ("error out"=w69:errorcluster, "Full Data (String) Out"=w70:string[][], "UEF Calculated Values Input out"=w72:T2)  [unwired: 6 in]
      n10 = call "HEWH Search for Bad Data.vi"("UEF Calculated Values Input"=w72, "Full DBL Array"=w65, "Full String Array"=w70, "error in (no error)"=w69) -> ("UEF Calculated Values Output"=w64:T2, "Full DBL Array Out"=w62:dbl[][], "Message String 1"=w73:string, "error out"=w66:errorcluster)  [unwired: 8 in]
      n11 = call "HEWH Find Bad Headers.vi"("Full Data (String)"=w60, "error in (no error)"=w66, "Message String 1"=w73, "UEF Calculated Values Input"=w64) -> ("error out"=w67:errorcluster, "UEF Calculated Values Output"=w74:T2)  [unwired: 6 in]
      n12 = call "HEWH Gas Type Detection.vi"("Full Data (String)"=w60, "error in (no error)"=w67, "UEF Calculated Values Input"=w74) -> ("error out"=w61:errorcluster, "UEF Calculated Values Output"=w63:T2)  [unwired: 7 in]
      n13 = call "HEWH Find Test Start Index.vi"("error in (no error)"=w61, "Full Data DBL"=w62, "UEF Calculated Values"=w63) -> ("error out"=w91:errorcluster, "Full Data DBL Out"=w88:dbl[][], "UEF Calculated Values Output"=w90:T2)  [unwired: 6 in]
      n14 = call "HEWH Find Test End Index.vi"("Test Type"=w12, "error in (no error)"=w91, "Full Data DBL"=w88, "UEF Calculated Values in"=w90) -> ("error out"=w89:errorcluster, "Full Data DBL Out"=w86:dbl[][], "UEF Calculated Values out"=w87:T2)  [unwired: 5 in]
      n15 = call "HEWH Find T0.vi"("Test Type"=w12, "Water Heater Type"=w19, "Error In"=w89, "Full Data DBL"=w86, "UEF Calculated Values"=w87) -> ("Error Out"=w77:errorcluster, "UEF Calculated Values (Output)"=w78:T2)  [unwired: 4 in, 1 out]
      n16 = call "HEWH Start Stop Index Array.vi"("Index Type"=HEWH_Index_Type."Draw Index", "error in (no error)"=w77, "UEF Calculated Values in"=w78) -> ("error out"=w83:errorcluster, "UEF Calculated Values Output"=w47:T2)  [unwired: 7 in]
      n17 = call "HEWH Extract Draw Data.vi"("Test Type"=w12, "error in (no error)"=w83, "UEF Calculated Values in"=w47) -> ("error out"=w49:errorcluster, "UEF Calculated Values Out"=w48:T2)  [unwired: 7 in]
      n18 = call "HEWH Non-Draw Index.vi"("error in (no error)"=w49, "UEF Calculated Values"=w48) -> ("error out"=w80:errorcluster, "UEF Calculated Values Output"=w79:T2)  [unwired: 8 in]
      n19 = call "HEWH Start Stop Index Array.vi"("Index Type"=HEWH_Index_Type."Heating Index", "error in (no error)"=w80, "UEF Calculated Values in"=w79) -> ("error out"=w75:errorcluster, "UEF Calculated Values Output"=w76:T2)  [unwired: 7 in]
      n20 = call "HEWH Extract First Hour Data DBL.vi"("error in (no error)"=w75, "UEF Calculated Values Input in"=w76) -> ("error out"=w94:errorcluster, "Upper Most Element"=w96:T9, "UEF Calculated Values Input out"=w95:T2)  [unwired: 7 in]
      n21 = call "HEWH Find Exact Cutout Location.vi"("error in (no error)"=w94, "Upper Most Element"=w96, "UEF Calculated Values Input in"=w95) -> ("error out"=w101:errorcluster, "Cut Out Location"=w97:dbl, "UEF Calculated Values Input in 2"=w98:T2)  [unwired: 6 in]
      n22 = call "Cutout Before 1 Hour Mark Check"("error in (no error)"=w101, "ExactCutout"=w97, "UEF Calculated Values Input in in"=w98) -> ("error out"=w102:errorcluster, "Output"=w99:i32, "UEF Calculated Values Output"=w100:T2)  [unwired: 6 in]
      n23 = case shown="0, Default" w99 {
        tunnel: w100 -> [w116 w120]
        tunnel: [w113 w119] -> w103
        tunnel: w102 -> [w114 w121]
        tunnel: [w112 w118] -> w104
        frame 0, Default {
          # "Vn is the draw that will have\na correction factor since you \ndid not make it at 1 hour\n\nNeeds cleaned up!"
          # "Forced Draw After 1 Hour"
          n24 = call "HEWH FHR Previous Temps.vi"("error in (no error)"=w114, "UEF Calculated Values Input"=w116) -> ("error out"=w115:errorcluster, "UEF Calculated Values Output"=w117:T2)  [unwired: 8 in]
          n25 = call "HEWH Find Vn.vi"("error in (no error)"=w115, "UEF Calculated Values Input"=w117) -> ("error out"=w112:errorcluster, "UEF Calculated Values Output"=w113:T2)  [unwired: 8 in]
        }
        frame 1 {
          # "No Forced Draw After 1 Hour"
          n26 = call "FHD No Forced Draw.vi"("error in (no error)"=w121, "UEF Calculated Values Output in"=w120) -> ("error out"=w118:errorcluster, "UEF Calculated Values Output out"=w119:T2)  [unwired: 8 in]
        }
      }
      n27 = call "HEWH FHD Category Determination.vi"("Water Heater Type"=w19, "error in (no error)"=w104, "UEF Calculated Values Input"=w103) -> ("error out"=w92:errorcluster, "UEF Calculated Values Output"=w93:T2)  [unwired: 7 in]
      n28 = call "HEWH Mass Removed.vi"("Error In"=w92, "UEF Calculated Values Output in"=w93) -> ("Error Out"=w33:errorcluster, "UEF Calculated Values Output out"=w34:T2)  [unwired: 8 in]
      n29 = call "HEWH Analyze Flow Rates.vi"("UEF Calculated Values Input"=w34, "Test Type"=w12, "error in (no error)"=w33) -> ("UEF Calculated Values Output"=w44:T2, "error out"=w43:errorcluster)  [unwired: 11 in]
      n30 = call "HEWH Analyze Total.vi"("Test Type"=w12, "error in (no error)"=w43, "UEF Calculated Values Input"=w44) -> ("error out"=w45:errorcluster, "UEF Calculated Values Output"=w46:T2)  [unwired: 7 in]
      n31 = call "HEWH Check Voltage.vi"("error in (no error)"=w45, "UEF Calculated Values Input"=w46) -> ("error out"=w35:errorcluster, "UEF Calculated Values Output"=w36:T2)  [unwired: 8 in]
      n32 = call "HEWH Check Ambient Temp.vi"("Water Heater Type"=w19, "error in (no error)"=w35, "UEF Calculated Values Input"=w36) -> ("error out"=w37:errorcluster, "UEF Calculated Values Output"=w40:T2)  [unwired: 7 in]
      n33 = call "HEWH Check Inlet Temps.vi"("error in (no error)"=w37, "UEF Calculated Values Input"=w40) -> ("error out"=w38:errorcluster, "UEF Calculated Values Output"=w41:T2)  [unwired: 8 in]
      n34 = call "HEWH Setpoint Temperature Test Requriments.vi"("error in"=w38, "UEF Calculated Values Input"=w41) -> ("error out"=w39:errorcluster, "UEF Calculated Values Output"=w42:T2)  [unwired: 8 in]
      n35 = call "HEWH Check Max Outlet Temp.vi"("Water Heater Type"=w19, "error in (no error)"=w39, "UEF Calculated Values Input"=w42) -> ("error out"=w32:errorcluster, "PercentInRange"=w13:dbl, "UEF Calculated Values Output"=w30:T2)  [unwired: 6 in]
      n36 = call "HEWH Compile Errors.vi"("error in (no error)"=w32, "UEF Calculated Values Input"=w30) -> ("error out"=w31:errorcluster, "UEF Calculated Values Output"=w29:T2)  [unwired: 8 in]
      n37 = call "HEWH Error Check.vi"("Test Type"=w12, "Water Heater Type"=w19, "error in (no error)"=w31, "UEF Calculated Values Output in"=w29) -> ("error out"=w17:errorcluster, "UEF Calculated Values Output"=w16:T2)  [unwired: 6 in]
      n38 = call "HEWH Info and Date.vi"("error in (no error)"=w17, "UEF Calculated Values Output in"=w16) -> ("error out"=w21:errorcluster, "UEF Calculated Values Output out"=w23:T2)  [unwired: 8 in]
      n39 = call "HEWH Spec Data.vi"("Water Heater Type"=w19, "Test Type"=w12, "error in (no error)"=w21, "UEF Calculated Values Input"=w23) -> ("error out"=w22:errorcluster, "UEF Calculated Values Output"=w24:T2)  [unwired: 6 in]
      n40 = call "HEWH Setpoint Info.vi"("error in (no error)"=w22, "UEF Calculated Values Input"=w24) -> ("error out"=w26:errorcluster, "UEF Calculated Values Output"=w27:T2)  [unwired: 8 in]
      n41 = call "FHR Header.vi"("error in (no error)"=w26, "UEF Calculated Values Input"=w27) -> ("error out"=w25:errorcluster, "UEF Calculated Values Output"=w28:T2, "First Hour Rating (Gallons)"=w18:dbl)  [unwired: 6 in, 1 out]
      n42 = call "HEWH Summary Error Check Data.vi"("Error In"=w25, "UEF Calculated Values Output in"=w28) -> ("Error Out"=w20:errorcluster, "UEF Calculated Values Output"=w15:T2)  [unwired: 8 in]
      n43 = call "HEWH Front Panel Display Indexer.vi"("Test Type"=w12, "Water Heater Type"=w19, "error in (no error)"=w20, "UEF Calculated Values Input"=w15) -> ("error out"=w105:errorcluster, "UEF Calculated Values Output"=w14:T2)  [unwired: 6 in]
    }
    frame True {
      w122 = 0.0 ("First Hour Rating (Gallons)")
    }
  }
  "FHD During 1 Hour Output" <- w2
  "FHD Full Data" <- w10
  "error out" <- w7
  "First Hour Rating (Gallons)" <- w3
  "PercentInRange" <- w1
  n44 = disable-structure shown="Disabled" {
    frame Disabled {
      w126 = TRUE  # DBL?
      # "Check for a valid test"
      # "Determine the usage pattern\nand check the draw count"
      # "Look for each draw\nthat has happened"
      # "Find all the data indexes"
      # "See if you get full or\npartial credit and apply\ncalculation"
      n45 = call "HEWH FHD Bonus.vi"() -> ()  [unwired: 10 in, 2 out]
      n46 = call "HEWH Header Length.vi"("DBL?"=w126) -> ()  [unwired: 7 in, 4 out]
      n47 = call "HEWH Extract Required Data.vi"() -> ()  [unwired: 9 in, 3 out]
      n48 = call "HEWH Water Properties Calculation.vi"() -> ()  [unwired: 10 in, 2 out]
      n49 = call "HEWH Usage Cluster.vi"() -> ()  [unwired: 10 in, 2 out]
      n50 = call "HEWH Find Test Start.vi"() -> ()  [unwired: 10 in, 2 out]
      n51 = call "HEWH Determine Data Type.vi"() -> ()  [unwired: 9 in, 3 out]
      n52 = call "HEWH Find Draw.vi"() -> ()  [unwired: 10 in, 2 out]
      n53 = call "HEWH Partial Credit Calc.vi"() -> ()  [unwired: 10 in, 2 out]
      n54 = call "HEWH Check Test Limits.vi"() -> ()  [unwired: 9 in, 3 out]
      n55 = call "HEWH FHR Headers.vi"() -> ()  [unwired: 8 in, 4 out]
    }
    frame Enabled {
    }
  }
